vi "Connect.vi"(0 "reference":refnum<class "VdTcpIP.lvclass">, 1 "timeout ms (60000)":i32=60000, 5 "error in (no error)":errorcluster) -> (14 "reference out":refnum<class "VdTcpIP.lvclass">, 15 "ConnectionExists":bool, 19 "error out":errorcluster)   [LabVIEW 2020, in "VdTcpIP.lvclass"]
doc: "Tries to connect"
uses:
  VdTcpIP.lvclass
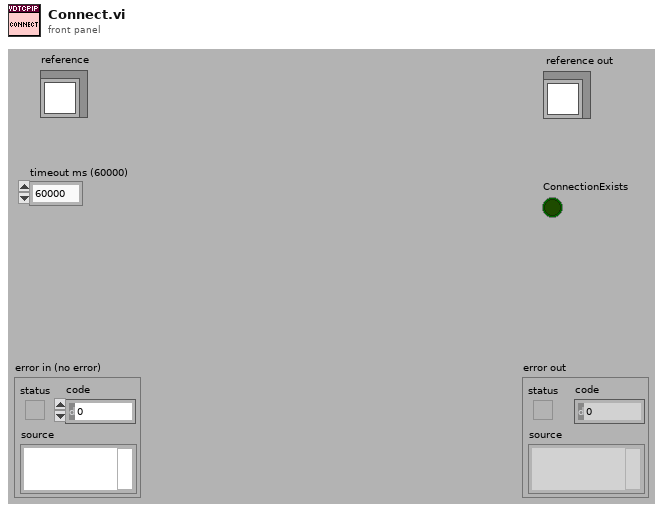
[diagram p1: front panel]
types:
  T1 = typedef "VdTcpIP.lvclass/ObjectAttributes.ctl" = cluster{"IP-Address":string, "Port":u16, "Connection":refnum<k5>, "Listener":refnum<k5>, "ListenerConnection":refnum<k5>, "Listner":bool, "ListnerProcessRunning":bool, "InConnections":refnum<k5>[], "InConnectionsIP":string[], "InConnectionAdded":refnum<notifier>, "RunVIOnNewConnection":variant, "DataToNewConnectionVI":cluster{"ControlName":string, "ControlValue":variant}[], "WebServicesURL_Location(http://...)":string, "WebServicesPostWebPage(*.asmx)":string, "Semaphore":T2, "AutoReConnectTimes":i32, "AutoReConnectInterval(ms)":i32, "ConnectionTimeout":i32}
  T2 = typedef "Semaphore RefNum" = refnum<k1>
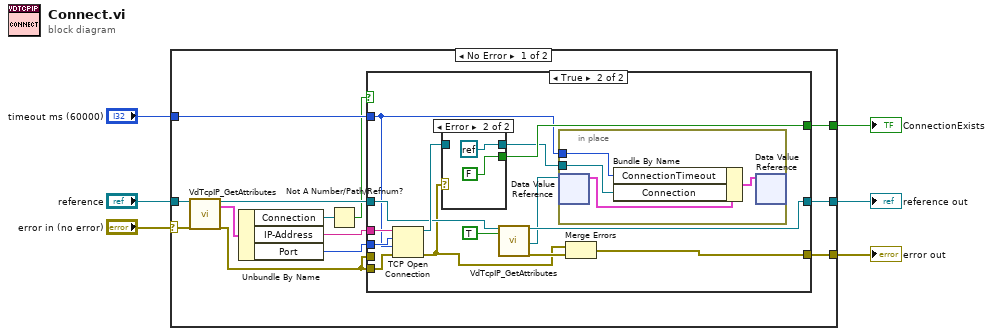
[diagram p0: block diagram]
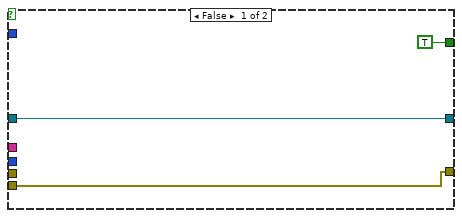
[diagram p2: hidden frame]
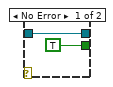
[diagram p3: hidden frame]
diagram:
  n1 = case shown="No Error" "error in (no error)" {
    selector: "error in (no error)" -> [w10 w45]
    tunnel: "reference" -> [w19 w46]
    tunnel: [w8 w45] -> w4
    tunnel: [w13 w46] -> w3
    tunnel: "timeout ms (60000)" -> [w16 _]
    tunnel: [w11 _] -> w1
    frame No Error {
      n2 = call "VdTcpIP_GetAttributes.vi"("reference in"=w19, "error in (no error)"=w10) -> ("reference out"=w14:refnum<class "VdTcpIP.lvclass">, "Data"=w7:T1, "error out"=w9:errorcluster)  [unwired: 1 in, 14 out]
      n3 = Unbundle By Name(w7) -> ("Connection"=w15:refnum<k5>, "IP-Address"=w18:string, "Port"=w17:u16)
      n4 = Not A Number/Path/Refnum?(number/path/refnum=w15) -> (NaN/Path/Refnum?=w12:bool)
      n5 = case shown="True" w12 {
        tunnel: w18 -> [_ w36]
        tunnel: w17 -> [_ w35]
        tunnel: w16 -> [_ w25]
        tunnel: w9 -> [w20 w30]
        tunnel: w14 -> [w22 w33]
        tunnel: [w22 w32] -> w13
        tunnel: [TRUE w31] -> w11
        tunnel: w9 -> [_ _]
        tunnel: [w20 w24] -> w8
        frame False {
        }
        frame True {
          n6 = TCP Open Connection(address=w36, remote port or service name=w35, timeout ms (60000)=w25, error in (no error)=w30) -> (connection ID=w34:refnum<k5>, error out=w23:errorcluster)  [unwired: 1 out]
          n7 = case shown="Error" w23 {
            tunnel: [w42 refnum<k0> refnum] -> w26
            tunnel: w34 -> [w42 _]
            tunnel: [TRUE FALSE] -> w31
            frame No Error {
            }
            frame Error {
            }
          }
          n8 = call "VdTcpIP_GetAttributes.vi"("reference in"=w33, "OnlyGetDvrReference(False)"=TRUE) -> ("reference out"=w32:refnum<class "VdTcpIP.lvclass">, "DataRef"=w27:refnum<data-value>, "error out"=w29:errorcluster)  [unwired: 14 in, 1 out]
          n9 = in-place {
            in-place-border: w26 -> [w39]
            in-place-border: w25 -> [w37]
            n10 = in-place-dvr #1(w27) -> (w40:T1)  [unwired: 1 out]
            n11 = Bundle By Name(cluster=w40, "ConnectionTimeout"=w37, "Connection"=w39) -> (w38:T1)
            n12 = in-place-dvr #1(w38) -> ()  [unwired: 2 out]
          }
          n13 = Merge Errors(w23, w29) -> (w24:errorcluster)
        }
      }
    }
    frame Error {
    }
  }
  "reference out" <- w3
  "error out" <- w4
  "ConnectionExists" <- w1
